vi "AMZ_S3_Create CanonicalizedResource String.vi"(10 "Bucket":string, 11 "Path and query string":string) -> (3 "Canonicalized Resource":string)   [LabVIEW 2015, in "LV Interface for Amazon S3.lvlib"]
doc: "Create the CanonicalizedResource part of the String to Sign."
uses:
  LV Interface for Amazon S3.lvlib
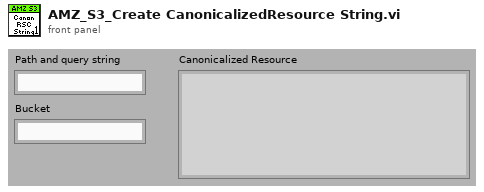
[diagram p1: front panel]
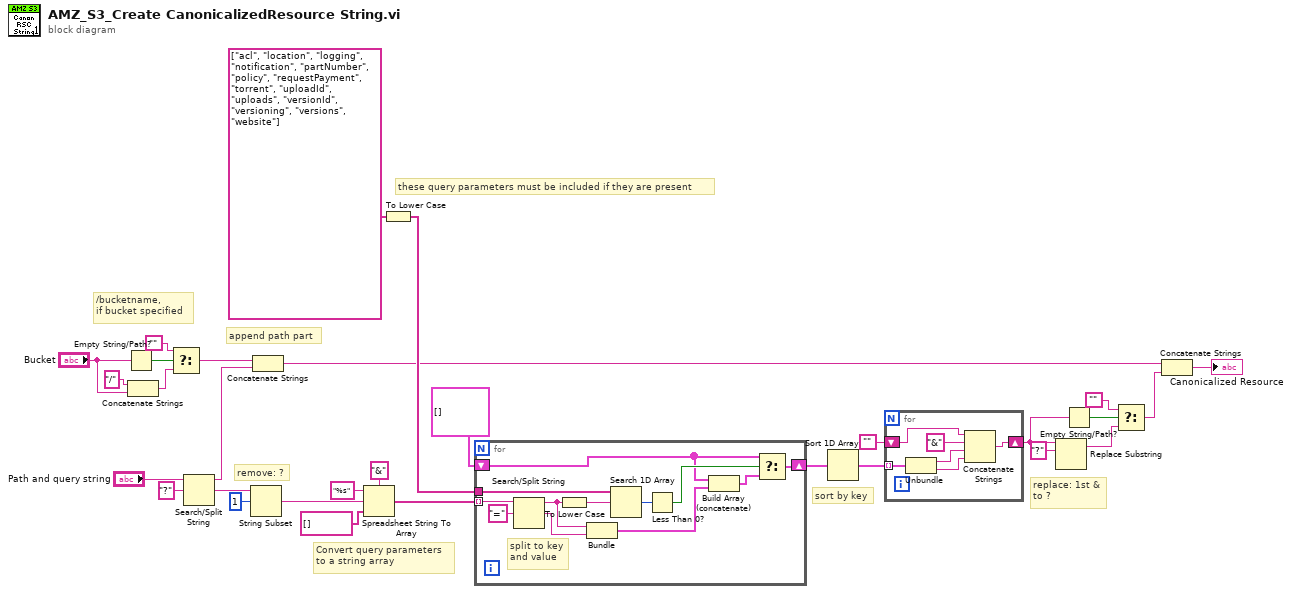
[diagram p0: block diagram]
diagram:
  # "Convert query parameters\nto a string array"
  # "these query parameters must be included if they are present"
  # "replace: 1st &\nto ?"
  # "sort by key"
  # "append path part"
  # "/bucketname,\nif bucket specified"
  # "remove: ?"
  n1 = Empty String/Path?(string/path="Bucket") -> (empty?=w30:bool)
  n2 = Concatenate Strings("/" ("string"), "Bucket") -> (w26:string)
  n3 = Select(t="", s=w30, f=w26) -> (s? t:f=w25:string)
  n4 = Search/Split String(string="Path and query string", search string/char (-)="?") -> (substring before match=w22:string, match + rest of string=w21:string)  [unwired: 1 in, 1 out]
  n5 = String Subset(string=w21, offset (0)=1) -> (substring=w19:string)  [unwired: 1 in]
  n6 = Concatenate Strings(w25, w22) -> (w8:string)
  n7 = Spreadsheet String To Array(delimiter (Tab)="&", format string="%s", spreadsheet string=w19, array type (2D Dbl)=string[] []) -> (array=w15:string[])
  n8 = To Lower Case(string=string[] ["acl", "location", "logging", "notification", "partNumber", "policy", "requestPayment", "torrent", "uploadId", "uploads", "versionId", "versioning", "versions", "website"]) -> (all lower case string=w13:string[])
  n9 = for {
    tunnel: w15 -> [w41] mode=indexing
    shift-right: [w32] -> w11
    shift-left: cluster{string, string}[] [] -> [w31]
    tunnel: w13 -> [w39]
    # "split to key\nand value"
    n10 = Search/Split String(string=w41, search string/char (-)="=") -> (substring before match=w36:string, match + rest of string=w35:string)  [unwired: 1 in, 1 out]
    n11 = To Lower Case(string=w36) -> (all lower case string=w40:string)
    n12 = Bundle(w36, w35) -> (w34:cluster{string, string})  [unwired: 1 in]
    n13 = Search 1D Array(1D array=w39, element=w40) -> (index of element=w38:i32)  [unwired: 1 in]
    n14 = Less Than 0?(x=w38) -> (x < 0?=w37:bool)
    n15 = Build Array (concatenate)(w31, w34) -> (w33:cluster{string, string}[])
    n16 = Select(t=w31, s=w37, f=w33) -> (s? t:f=w32:cluster{string, string}[])
  }
  n17 = Sort 1D Array(array=w11) -> (sorted array=w10:cluster{string, string}[])
  n18 = for {
    tunnel: w10 -> [w48] mode=indexing
    shift-right: [w45] -> w5
    shift-left: "" -> [w43]
    n19 = Unbundle(w48) -> (w47:string, w46:string)
    n20 = Concatenate Strings(w43, "&" ("string"), w47, w46) -> (w45:string)
  }
  n21 = Replace Substring(4:"?" ("substring (\"\")"), 5:w5) -> (1:w3:string)  [unwired: 2 in, 1 out]
  n22 = Empty String/Path?(string/path=w5) -> (empty?=w4:bool)
  n23 = Select(t="", s=w4, f=w3) -> (s? t:f=w2:string)
  n24 = Concatenate Strings(w8, w2) -> (→"Canonicalized Resource":string)
